vi "Control Panel.vi"(8 "error in (no error)":errorcluster, 11 "fake Laser Power Controller in":refnum<class "Laser Power Controller.lvclass">) -> (0 "error out":errorcluster, 3 "fake Laser Power Controller out":refnum<class "Laser Power Controller.lvclass">)   [LabVIEW 2009, in "Laser Power Controller.lvclass"]
doc: "(Dynamic) A user-level application that simulates the physical front panel of the Instrument. Provide the user with buttons to manually control features of the instrument, and provide indicators of its current state."
uses:
  Laser Power Controller.lvclass
  Utility Classes/Scannable/Scannable.lvclass
  Laser Power Controller.lvclass/Laser Power Controller.ctl
  BEOC LPC/BEOC LPC.lvlib
panel:
  in  "Set":bool
  in  "Read to Control":bool
  in  "Read":bool
  in  "Copy actual to set":bool
  in  "Populate fields with member data":bool
  out "front-panel controls":enum16{"enabled", "disabled"}(ring)
  out "control mode":T1(ring)
  out "wavelength":dbl[unit]
  out "power":dbl[unit]
  in  "front-panel controls set":enum16{"enabled", "disabled"}(ring)
  in  "control mode set":T1(ring)
  in  "wavelength set":dbl[unit]=8.300000000000001e-07
  in  "power set":dbl[unit]=0.005
  in  "stop":bool
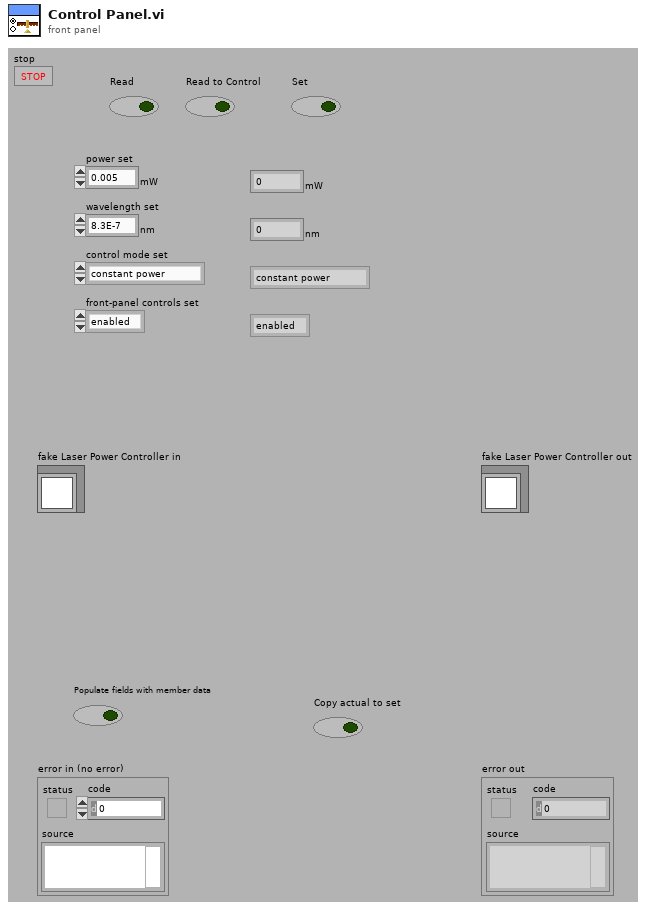
[diagram p1: front panel]
types:
  T1 = enum16{"constant power", "constant transmission"}
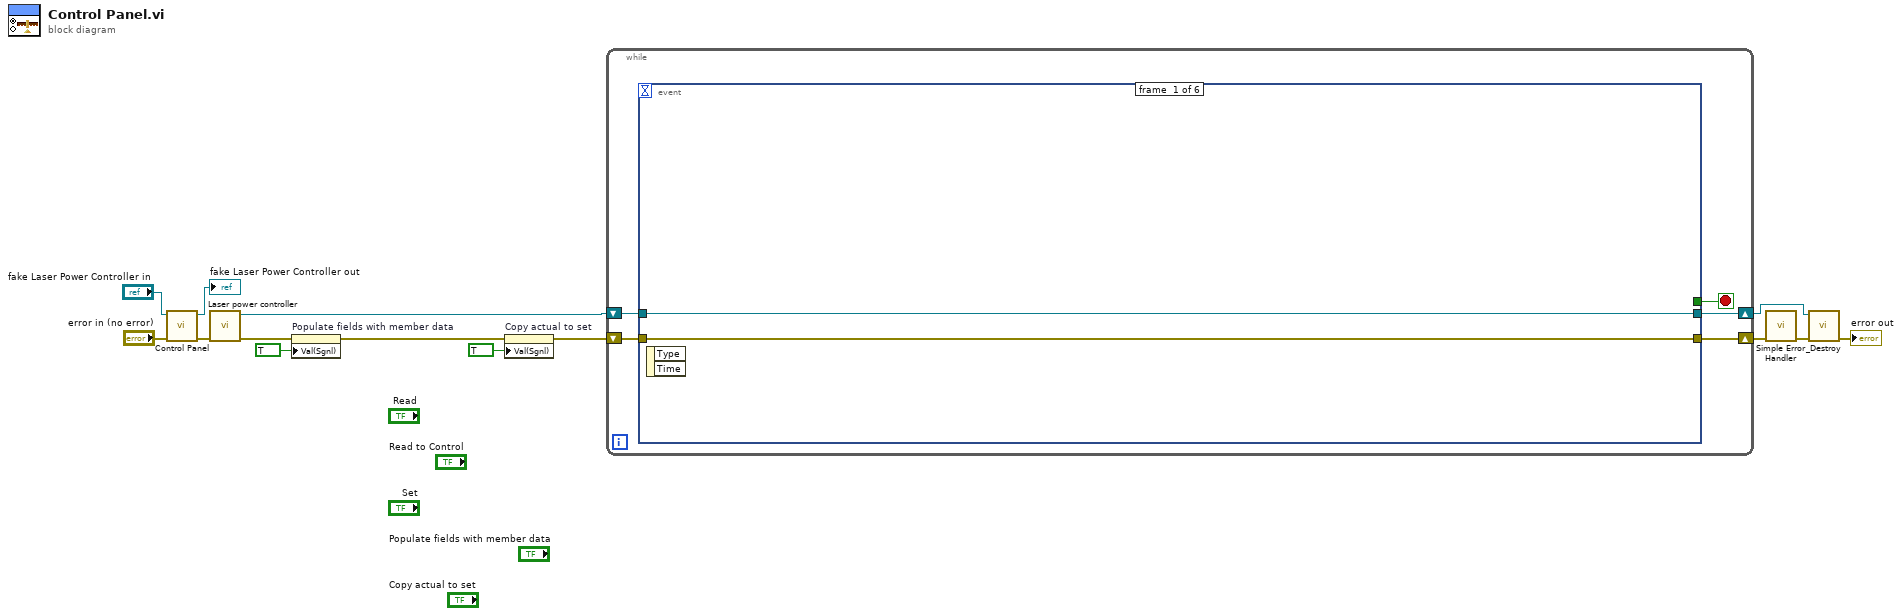
[diagram p0: block diagram]
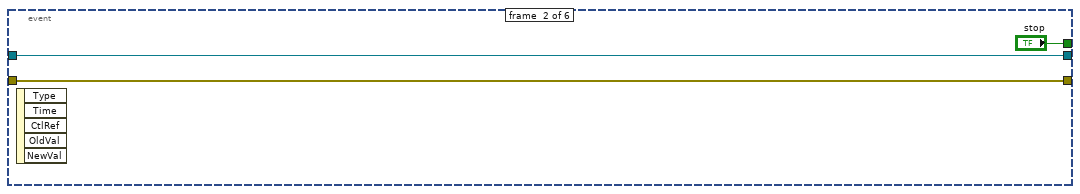
[diagram p2: hidden frame]
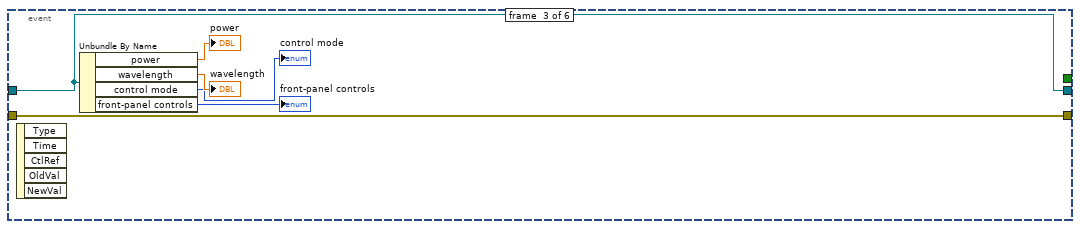
[diagram p3: hidden frame]
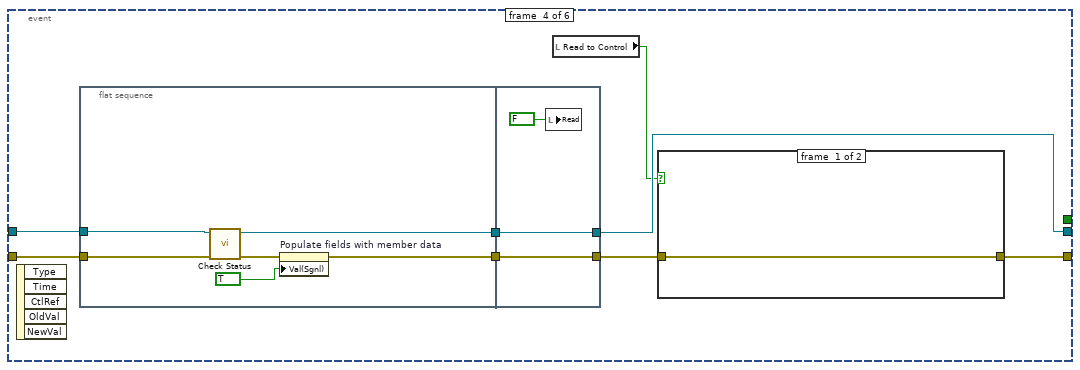
[diagram p4: hidden frame]
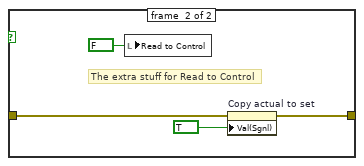
[diagram p5: hidden frame]
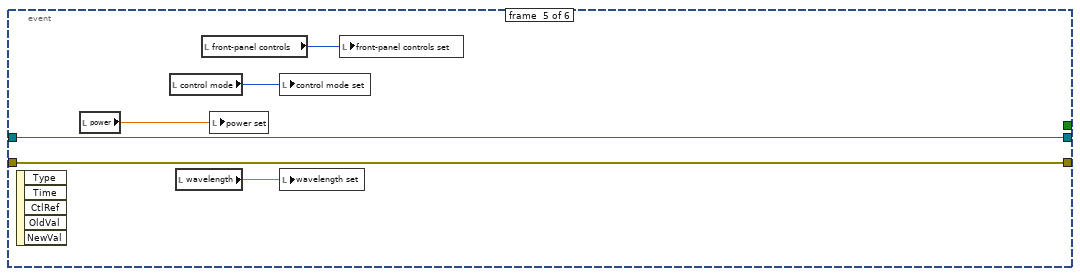
[diagram p6: hidden frame]
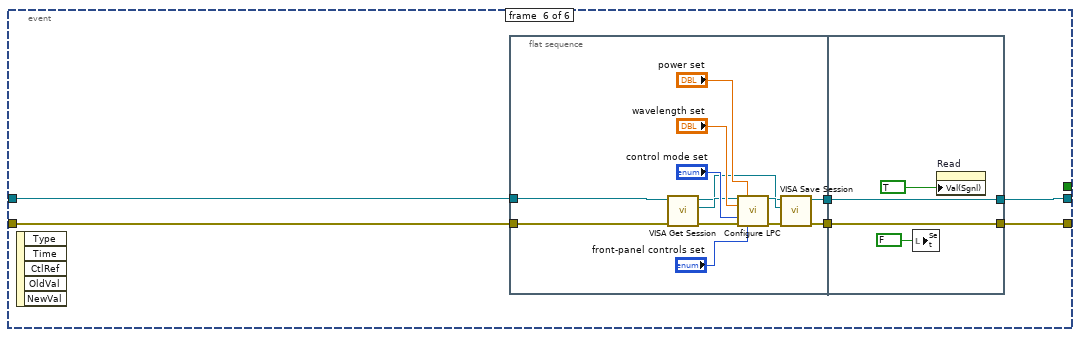
[diagram p7: hidden frame]
diagram:
  n1 = call-parent "Control Panel.vi"("error in (no error)"="error in (no error)", "Instrument in"="fake Laser Power Controller in") -> ("error out"=w10:errorcluster, "Instrument out"=→"fake Laser Power Controller out":refnum<class "Laser Power Controller.lvclass">)  [unwired: 8 in]
  n2 = call "Laser power controller.vi"("error in (no error)"=w10) -> ("error out"=w9:errorcluster, "Laser Power Controller out"=w6:refnum<class "Laser Power Controller.lvclass">)  [unwired: 9 in]
  n3 = property on="Populate fields with member data" class="Bool (strict)"(error in=w9, "Val(Sgnl)"=TRUE ("Value (Signaling)")) -> (error out=w8:errorcluster)  [unwired: 1 in, 1 out]
  n4 = property on="Copy actual to set" class="Bool (strict)"(error in=w8, "Val(Sgnl)"=TRUE ("Value (Signaling)")) -> (error out=w3:errorcluster)  [unwired: 1 in, 1 out]
  n5 = while {
    shift-right: [w16] -> w2
    shift-left: w6 -> [w18]
    shift-right: [w15] -> w1
    shift-left: w3 -> [w17]
    stop <- w19 stop-if-true
    n6 = event shown="[5] \"Set\": Value Change" {
      selector: _ -> [_ _ _ _ _ _]
      dyn-events: _ -> [_ _ _ _ _ _]
      timeout: _ -> [_ _ _ _ _ _]
      tunnel: [_ "stop" _ _ _ _] -> w19
      tunnel: w18 -> [w20 w23 w29 w38 w57 w64]
      tunnel: [w20 w23 w29 w37 w57 w63] -> w16
      tunnel: w17 -> [w21 w22 w30 w34 w58 w62]
      tunnel: [w21 w22 w30 w31 w58 w61] -> w15
      event #0 {
        n7 = event-data() -> ()  [unwired: 1 in, 2 out]
      }
      event #1 {
        n8 = event-data() -> ()  [unwired: 1 in, 5 out]
      }
      event #2 {
        n9 = event-data() -> ()  [unwired: 1 in, 5 out]
        n10 = Unbundle By Name(w29) -> ("power"=→"power":dbl[unit], "wavelength"=→"wavelength":dbl[unit], "control mode"=→"control mode":T1, "front-panel controls"=→"front-panel controls":enum16{"enabled", "disabled"})
      }
      event #3 {
        n11 = event-data() -> ()  [unwired: 1 in, 5 out]
        n12 = flat-sequence {
          tunnel: w38 -> [w48]
          tunnel: [w47] -> w36
          tunnel: w34 -> [w45]
          tunnel: [w44] -> w32
          tunnel: [w52] -> w37
          tunnel: w36 -> [w52]
          tunnel: [w50] -> w33
          tunnel: w32 -> [w50]
          frame #0 {
            n13 = call-dynamic "Check Status.vi"("error in (no error)"=w45, "Laser Power Controller in"=w48) -> ("error out"=w46:errorcluster, "Laser Power Controller out"=w47:refnum<class "Laser Power Controller.lvclass">)  [unwired: 6 in, 2 out]
            n14 = property on="Populate fields with member data" class="Bool (strict)"(error in=w46, "Val(Sgnl)"=TRUE ("Value (Signaling)")) -> (error out=w44:errorcluster)  [unwired: 1 in, 1 out]
          }
          frame #1 {
            n15 = local write "Read"(FALSE ("Read")) -> ()
          }
        }
        n16 = local read "Read to Control"() -> (w35:bool)
        n17 = case shown="True" w35 {
          tunnel: w33 -> [w39 w41]
          tunnel: [w39 w40] -> w31
          frame #0 {
          }
          frame #1 {
            # "The extra stuff for Read to Control"
            n18 = local write "Read to Control"(FALSE ("Read to Control")) -> ()
            n19 = property on="Copy actual to set" class="Bool (strict)"(error in=w41, "Val(Sgnl)"=TRUE ("Value (Signaling)")) -> (error out=w40:errorcluster)  [unwired: 1 in, 1 out]
          }
        }
      }
      event #4 {
        n20 = event-data() -> ()  [unwired: 1 in, 5 out]
        n21 = local read "power"() -> (w56:dbl[unit])
        n22 = local read "control mode"() -> (w54:T1)
        n23 = local read "wavelength"() -> (w55:dbl[unit])
        n24 = local read "front-panel controls"() -> (w53:enum16{"enabled", "disabled"})
        n25 = local write "power set"(w56) -> ()
        n26 = local write "control mode set"(w54) -> ()
        n27 = local write "wavelength set"(w55) -> ()
        n28 = local write "front-panel controls set"(w53) -> ()
      }
      event #5 {
        n29 = event-data() -> ()  [unwired: 1 in, 5 out]
        n30 = flat-sequence {
          tunnel: w64 -> [w71]
          tunnel: w62 -> [w68]
          tunnel: [w70] -> w60
          tunnel: [w65] -> w59
          tunnel: [w80] -> w61
          tunnel: [w81] -> w63
          tunnel: w60 -> [w81]
          tunnel: w59 -> [w80]
          frame #0 {
            n31 = call-dynamic "VISA Get Session.vi"("error in (no error)"=w68, "Instrument.lvclass in"=w71) -> ("error out"=w67:errorcluster, "VISA Resource Name"=w73:refnum<visa-resource-name>, "Instrument.lvclass out"=w69:refnum<class "Laser Power Controller.lvclass">)  [unwired: 7 out]
            n32 = call "Configure LPC.vi"("VISA resource name"=w73, "power"="power set", "wavelength"="wavelength set", "control mode"="control mode set", "error in (no error)"=w67, "front-panel controls"="front-panel controls set") -> ("VISA resource name out"=w72:refnum<visa-resource-name>, "error out"=w66:errorcluster)  [unwired: 8 in]
            n33 = call-dynamic "VISA Save Session.vi"("error in (no error)"=w66, "VISA Resource Name"=w72, "Instrument.lvclass in"=w69) -> ("error out"=w65:errorcluster, "Instrument.lvclass out"=w70:refnum<class "Laser Power Controller.lvclass">)  [unwired: 7 out]
          }
          frame #1 {
            n34 = local write "Set"(FALSE ("Set")) -> ()
            n35 = property on="Read" class="Bool (strict)"("Val(Sgnl)"=TRUE ("Value (Signaling)")) -> ()  [unwired: 2 in, 2 out]
          }
        }
      }
    }
  }
  n36 = call <vilib>:"Simple Error Handler.vi"("error in (no error)"=w1) -> ("error out"=w4:errorcluster)  [unwired: 1 in, 7 out]
  n37 = call-dynamic "_Destroy.vi"("error in (no error)"=w4, "Instrument in"=w2) -> ("error out"=→"error out":errorcluster)  [unwired: 9 out]
